vi "cw_1.vi"() -> ()   [LabVIEW 2022 SP3]
doc: "Use this template to build a producer/consumer design pattern. Use this template when you need to execute a process, such as data analysis, when a data source, such as a triggered acquisition, produces data at an uneven rate and you need to execute the process when the data becomes available."
panel:
  out "# elements in queue":i32
  out "Measured Signal":dbl(graph)
  out "filtered signal":dbl(graph)
  in  "stop":bool
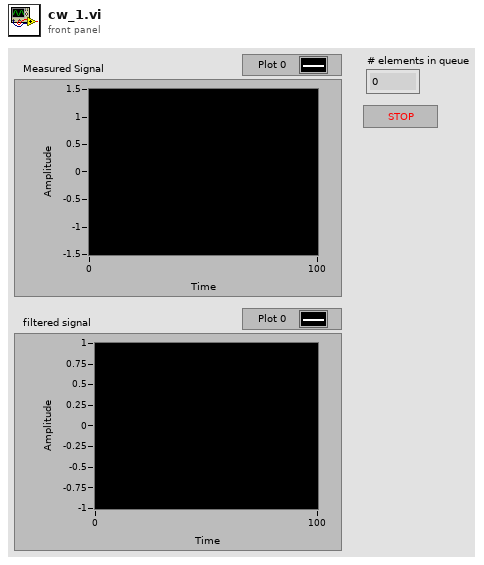
[diagram p1: front panel]
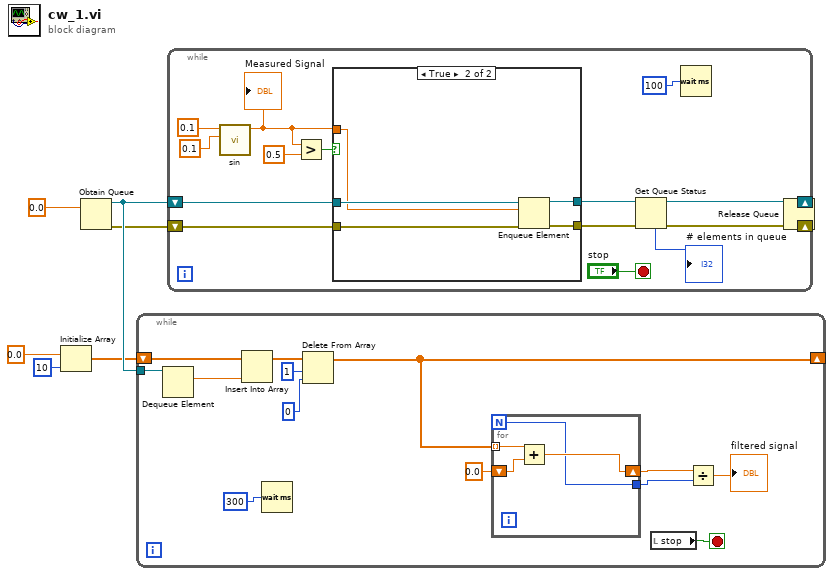
[diagram p0: block diagram]
diagram:
  n1 = Initialize Array(0.0, 10 ("dimension size")) -> (w1:dbl[])
  n2 = Obtain Queue(element data type=0.0) -> (queue out=w8:refnum<queue>, error out=w7:errorcluster)  [unwired: 4 in, 1 out]
  n3 = while {
    tunnel: w8 -> [w21]
    shift-right: [w15] -> _
    shift-left: w1 -> [w19]
    stop <- w9 stop-if-true
    n4 = Dequeue Element(queue=w21) -> (element=w20:dbl)  [unwired: 2 in, 3 out]
    n5 = Insert Into Array(array=w19, new element=w20) -> (w18:dbl[])  [unwired: 1 in]
    n6 = Wait (ms)(milliseconds to wait=u32 300) -> ()  [unwired: 1 out]
    n7 = Delete From Array(array=w18, length=1, index=0) -> (array with subset deleted=w15:dbl[])  [unwired: 1 out]
    n8 = for {
      N -> [w22]
      tunnel: w15 -> [w25] mode=indexing
      shift-right: [w24] -> w12
      shift-left: 0.0 -> [w23]
      tunnel: [w22] -> w11
      n9 = Add(x=w25, y=w23) -> (x+y=w24:dbl)
    }
    n10 = local read "stop"() -> (w9:bool)
    n11 = Divide(x=w12, y=w11) -> (x/y=→"filtered signal":dbl)
  }
  n12 = while {
    shift-right: [w27] -> w5
    shift-left: w7 -> [w37]
    shift-right: [w29] -> w6
    shift-left: w8 -> [w38]
    stop <- "stop" stop-if-true
    n13 = call "sin.vi"("noise amplitude"=0.1 ("dx"), "dx"=0.1) -> ("sin x"=w33:dbl)  [unwired: 8 in, 1 out]
    "Measured Signal" <- w33
    n14 = Greater?(x=w33, y=0.5) -> (0:w31:bool)
    n15 = case shown="True" w31 {
      tunnel: w38 -> [w41 w46]
      tunnel: [w41 w45] -> w30
      tunnel: w37 -> [w40 w44]
      tunnel: [w40 w43] -> w28
      tunnel: w33 -> [_ w42]
      frame False {
      }
      frame True {
        n16 = Enqueue Element(queue=w46, element=w42, error in (no error)=w44) -> (queue out=w45:refnum<queue>, error out=w43:errorcluster)  [unwired: 1 in, 1 out]
      }
    }
    n17 = Get Queue Status(queue=w30, error in (no error)=w28) -> (queue out=w29:refnum<queue>, error out=w27:errorcluster, # elements in queue=→"# elements in queue":i32)  [unwired: 1 in, 5 out]
    n18 = Wait (ms)(milliseconds to wait=u32 100) -> ()  [unwired: 1 out]
  }
  n19 = Release Queue(queue=w6, error in (no error)=w5) -> ()  [unwired: 1 in, 3 out]
